vi "Local adress check stm.vi"() -> ()   [LabVIEW 2017]
uses:
  <vilib>/Plasmionique/MB Master/MB_Master_Serial/MB_Master_Serial.lvclass
  D:/Program Files (x86)/National Instruments/LabVIEW 2017/vi.lib/Plasmionique/MB Master/MB_Master/MB_Master.lvclass
  <vilib>/Plasmionique/MB Master/MB Master.lvlib
panel:
  out "Registers":u16[](array[numeric])
  out "Error out":errorcluster
  out "code":i32
  in  "VISA Resource":refnum<visa-resource-name>="COM8"
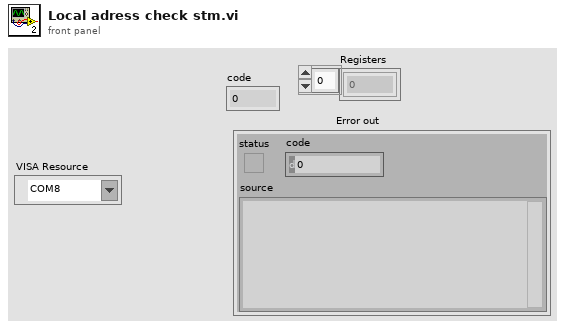
[diagram p1: front panel]
types:
  T1 = cluster{"baud rate (bps)":u32, "stop bits":u16, "parity":u16, "flow control":u16, "timeout":u32, "retries":i32}
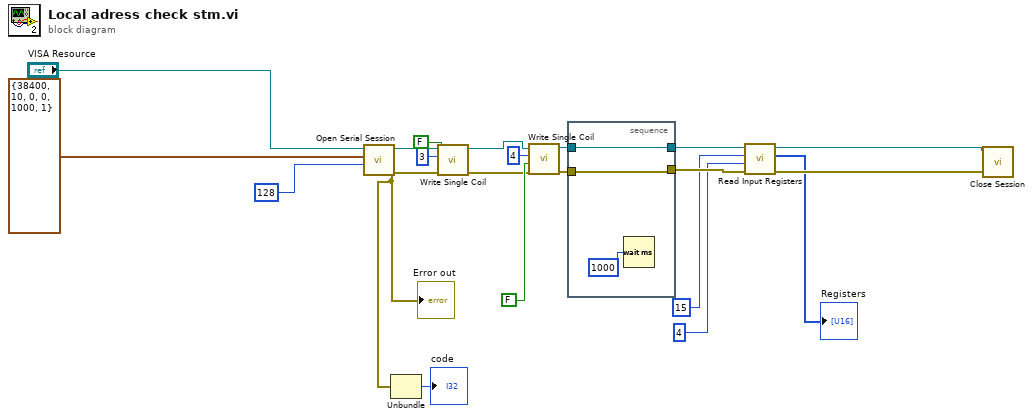
[diagram p0: block diagram]
diagram:
  n1 = call <vilib>:"Open Serial Session.vi"("Slave ID"=u8 128, "Serial Config"=T1 {"baud rate (bps)"=38400, "stop bits"=10, "parity"=0, "flow control"=0, "timeout"=1000, "retries"=1}, "VISA Resource"="VISA Resource") -> ("Error out"=w10:errorcluster, "MB_Serial session"=w11:refnum<class "MB_Master_Serial.lvclass">)  [unwired: 7 in]
  "Error out" <- w10
  n2 = Unbundle(w10) -> ("code"=→"code":i32)  [unwired: 2 out]
  n3 = call <vilib>:"Write Single Coil.vi"("error in (no error)"=w10, "value"=FALSE, "address"=u16 3, "MB session in"=w11) -> ("error out"=w12:errorcluster, "MB session out"=w13:refnum<class "MB_Master_Serial.lvclass">)  [unwired: 6 in]
  n4 = call <vilib>:"Write Single Coil.vi"("error in (no error)"=w12, "value"=FALSE, "address"=u16 4, "MB session in"=w13) -> ("error out"=w14:errorcluster, "MB session out"=w15:refnum<class "MB_Master_Serial.lvclass">)  [unwired: 6 in]
  n5 = stacked-sequence {
    tunnel: [w23] -> w7
    tunnel: w15 -> [w23]
    tunnel: [w22] -> w4
    tunnel: w14 -> [w22]
    frame #0 {
      n6 = Wait (ms)(milliseconds to wait=u32 1000) -> ()  [unwired: 1 out]
    }
  }
  n7 = call <vilib>:"Read Input Registers.vi"("error in (no error)"=w4, "quantity"=u16 4, "starting address"=u16 15, "MB session in"=w7) -> ("error out"=w5:errorcluster, "Registers"=→"Registers":u16[], "MB session out"=w6:refnum<class "MB_Master_Serial.lvclass">)  [unwired: 5 in]
  n8 = call-dynamic "Close Session.vi"("error in (no error)"=w5, "MB_Serial session"=w6) -> ()  [unwired: 9 in, 1 out]
